vi "gun_speed_test_feed_forward.vi"() -> ()   [LabVIEW 2011]
panel:
  out "XY Graph":cluster{dbl[], dbl[]}[](graph)
  in  "max":dbl
  in  "step":dbl
  in  "initial":dbl
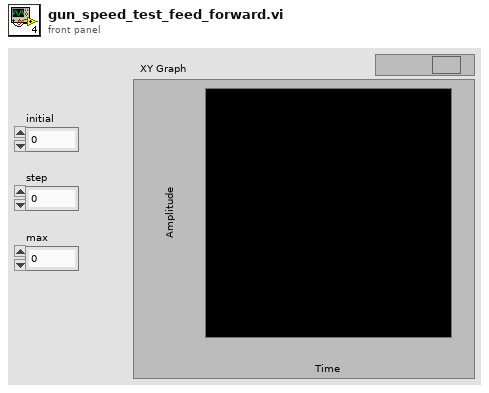
[diagram p1: front panel]
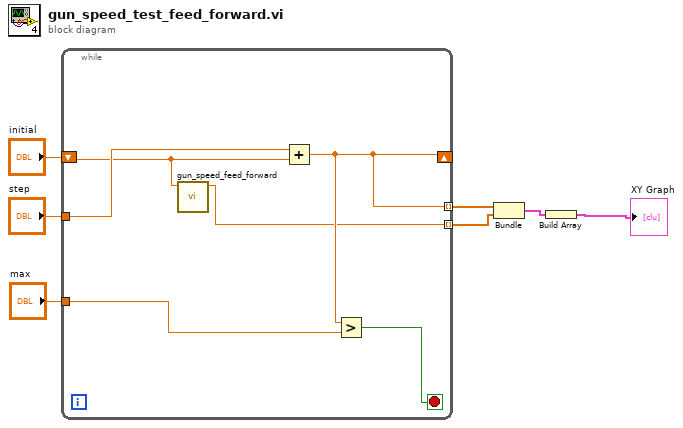
[diagram p0: block diagram]
diagram:
  n1 = while {
    shift-right: [w9] -> _
    shift-left: "initial" -> [w12]
    tunnel: "step" -> [w13]
    tunnel: "max" -> [w11]
    tunnel: [w9] -> w4 mode=indexing
    tunnel: [w8] -> w3 mode=indexing
    stop <- w10 stop-if-true
    n2 = call "gun_speed_feed_forward.vi"("RPM"=w12) -> ("Power"=w8:dbl)  [unwired: 10 in]
    n3 = Add(x=w13, y=w12) -> (x+y=w9:dbl)
    n4 = Greater?(x=w9, y=w11) -> (0:w10:bool)
  }
  n5 = Bundle(w4, w3) -> (w2:cluster{dbl[], dbl[]})  [unwired: 1 in]
  n6 = Build Array(w2) -> (→"XY Graph":cluster{dbl[], dbl[]}[])
